vi "MGCC_MdlMgmt_main.vi"() -> ()   [LabVIEW 2016]
doc: "-----------------------------------------------------------------------------------------------------------------------\nCopyright <2019> <The University of Tennessee at Knoxville and the University of Tennessee Research Foundation>\nThis software is released under BSD-3 \nhttps://opensource.org/licenses/BSD-3-Clause \nAdditional license options available at https://utrf.tennessee.edu/industry/sample-agreements/\n-----------------------------------------------------------------------------------------------------------------------\n\nThis VI is the main VI for the model management function. The main purpose of this VI is to initize the input for the state estimation and PQ balancing. Since it will only be run one time, there is no need for the enable button."
uses:
  Communication/MGCC_Global_communication_inputsettings .vi
  Data logging/Sub-Vis/Global tdms reference.vi
  Data logging/Sub-Vis/MGCC_DataLog_global.vi
  Communication/Global communication output.vi
  Communication/Global communication.vi
  Global_MdlMgmt.vi
  Resynchronization/MGCC_Resync_global.vi
  Islanded Control/MGCC_IsdCon_global1.vi
  Abnormal Fault State Control/Sub_VIs/Fault_Abnormal_state.vi
  <vilib>/imath/engines/lvmath2/RunTimeEngine/ErrorHandling/NIMS_Finalize Error.vi
  <vilib>/imath/engines/lvmath2/RunTimeEngine/BuiltInFunctions/double/NIMS_double.vi
  <vilib>/imath/engines/lvmath2/RunTimeEngine/NodeEndStatement/NIMS_NodeEndStatement_Output.vi
panel:
  out "x 2":dbl[][](array[numeric])
  out "x":dbl[][](array[numeric])
  out "appended array":dbl[](array[numeric])
  out "error out 4":errorcluster
  out "error out 3":errorcluster
  out "error out 2":errorcluster
  out "PV_hist":dbl[](array[numeric])
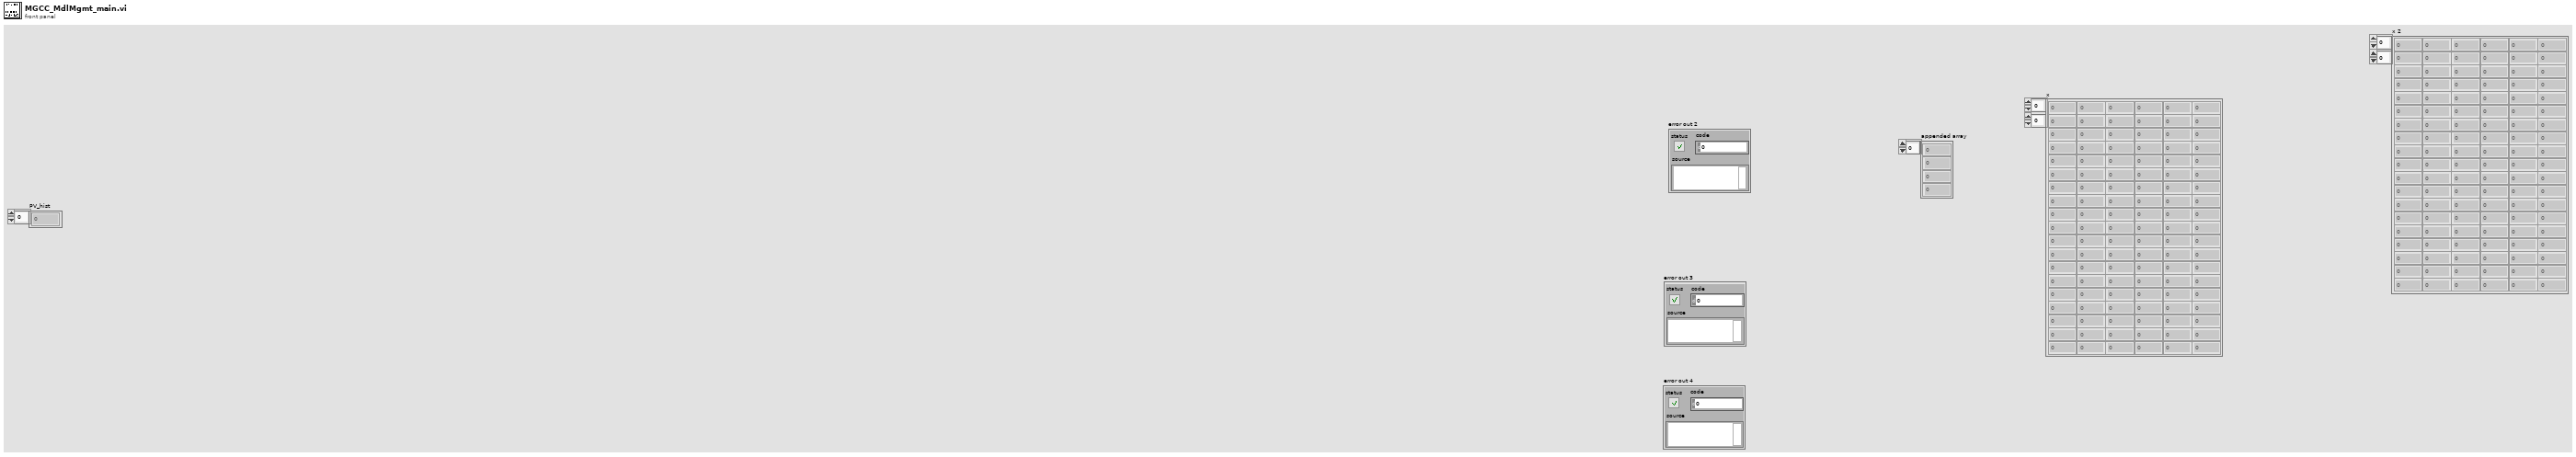
[diagram p1: front panel]
types:
  T1 = enum16{"open", "open or create", "create or replace", "create", "open (read-only)"}
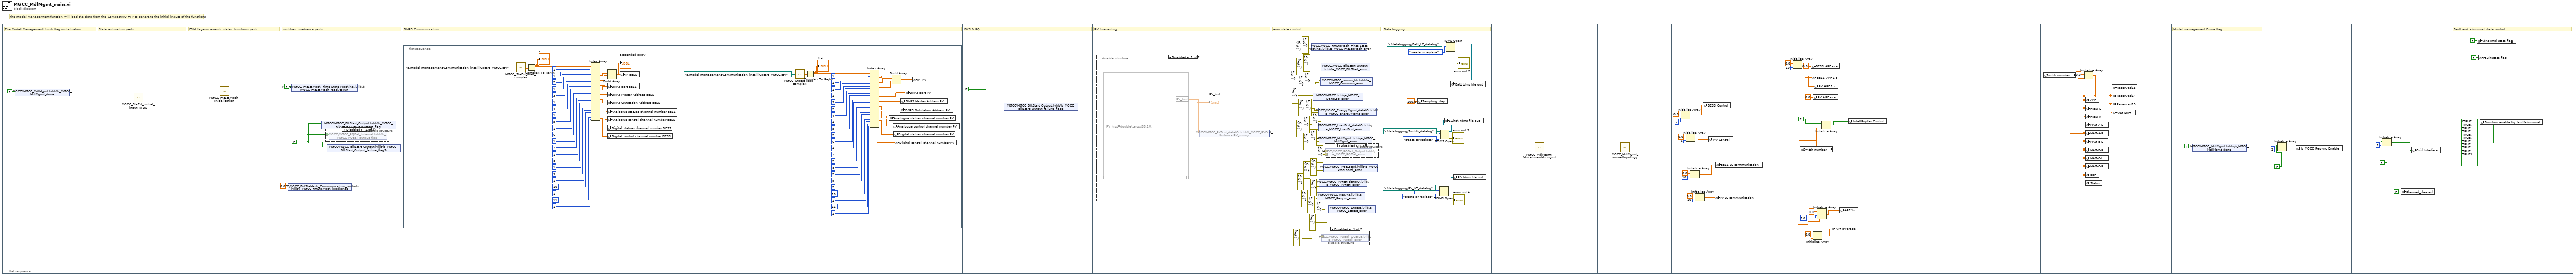
[diagram p0: block diagram]
diagram:
  # "the model management function will load the data from the CompactRIO FTP to generate the initial inputs of the functions"
  n1 = flat-sequence {
    frame #0 {
      # "The Model Management finish flag initialization"
      n2 = shared-variable "MGCC\\MGCC_MdlMgmt.lvlib\\b_MGCC_MdlMgmt_done"(FALSE ("b_MGCC_MdlMgmt_done")) -> ()  [unwired: 1 in, 1 out]
    }
    frame #1 {
      # "State estimation parts"
      n3 = call "MGCC_StaEst_initial_input_RTDS.vi"() -> ()  [unwired: 12 in]
    }
    frame #2 {
      # "FSM flagesm events, states, functions parts"
      n4 = call "MGCC_FntStaMach_Initialization.vi"() -> ()  [unwired: 12 in]
    }
    frame #3 {
      w2 = FALSE ("S0102-status-ctrl")
      # "switches, irradiance parts"
      n5 = shared-variable "MGCC\\MGCC_FntStaMach_Communication_controls.lvlib\\i_MGCC_FntStaMach_irradiance"(0.0 ("i_MGCC_FntStaMach_irradiance")) -> ()  [unwired: 1 in, 1 out]
      n6 = shared-variable "MGCC\\MGCC_FntStaMach_Finte State Machine.lvlib\\b_MGCC_FntStaMach_readytorun"(FALSE ("b_MGCC_FntStaMach_readytorun")) -> ()  [unwired: 1 in, 1 out]
      n7 = shared-variable "MGCC\\MGCC_BlkStart_Output.lvlib\\b_MGCC_BlkStart_Output_success_flag"(w2) -> ()  [unwired: 1 in, 1 out]
      n8 = disable-structure shown="Disabled" {
        disable-tunnel: w2 -> [w5 _]
        frame Disabled {
          n9 = shared-variable "MGCC\\MGCC_PQBal_Internal.lvlib\\b_MGCC_PQBal_output_flag"(w5) -> ()  [unwired: 1 in, 1 out]
        }
        frame Enabled {
        }
      }
      n10 = shared-variable "MGCC\\MGCC_BlkStart_Output.lvlib\\b_MGCC_BlkStart_Output_failure_flag5"(w2) -> ()  [unwired: 1 in, 1 out]
    }
    frame #4 {
      # "DNP3 Communication"
      n11 = flat-sequence {
        frame #0 {
          n12 = call "MGCC_StaEst_load_complex.vi"("file path (dialog if empty)"=path "c:/model-management/Communication_intellirupters_MGCC.csv" ("file path (use dialog)")) -> ("Array 13"=w29:cdb[][])
          n13 = Complex To Re/Im(x + iy=w29) -> (x=w28:dbl[][])  [unwired: 1 out]
          "x" <- w28
          n14 = Index Array(array=w28, index (row) #1=1 ("index (row)"), index (col) #1=1 ("disabled index (col)"), index (row) #2=2 ("index (row)"), index (col) #2=1 ("disabled index (col)"), index (row) #3=3 ("index (row)"), index (col) #3=1 ("disabled index (col)"), index (row) #4=4 ("index (row)"), index (col) #4=1 ("disabled index (col)"), index (row) #5=5 ("index (row)"), index (col) #5=1 ("disabled index (col)"), index (row) #6=6 ("index (row)"), index (col) #6=1 ("disabled index (col)"), index (row) #7=7 ("index (row)"), index (col) #7=1 ("disabled index (col)"), index (row) #8=8 ("index (row)"), index (col) #8=1 ("disabled index (col)"), index (row) #9=9 ("index (row)"), index (col) #9=1 ("disabled index (col)"), index (row) #10=10 ("index (row)"), index (col) #10=1 ("disabled index (col)"), index (row) #11=11 ("index (row)"), index (col) #11=1 ("disabled index (col)")) -> (element #1=w39:dbl, element #2=w32:dbl, element #3=w31:dbl, element #4=w30:dbl, element #5=w12:dbl, element #6=w11:dbl, element #7=w10:dbl, element #8=w9:dbl, element #9=w8:dbl, element #10=w7:dbl, element #11=w6:dbl)
          n15 = Build Array(w39, w32, w31, w30) -> (w13:dbl[])
          "appended array" <- w13
          n16 = global write "MGCC_Global_communication_inputsettings .vi" "DNP3 port BESS"(w12) -> ()
          n17 = global write "MGCC_Global_communication_inputsettings .vi" "DNP3 Master Address BESS"(w11) -> ()
          n18 = global write "MGCC_Global_communication_inputsettings .vi" "DNP3 Outstation Address BESS"(w10) -> ()
          n19 = global write "MGCC_Global_communication_inputsettings .vi" "Analogue statues channel number BESS"(w9) -> ()
          n20 = global write "MGCC_Global_communication_inputsettings .vi" "Analogue control channel number BESS"(w8) -> ()
          n21 = global write "MGCC_Global_communication_inputsettings .vi" "Digital statues channel number BESS"(w7) -> ()
          n22 = global write "MGCC_Global_communication_inputsettings .vi" "Digital control channel number BESS"(w6) -> ()
          n23 = global write "MGCC_Global_communication_inputsettings .vi" "IP_BESS"(w13) -> ()
        }
        frame #1 {
          n24 = call "MGCC_StaEst_load_complex.vi"("file path (dialog if empty)"=path "c:/model-management/Communication_intellirupters_MGCC.csv" ("file path (use dialog)")) -> ("Array 13"=w70:cdb[][])
          n25 = Complex To Re/Im(x + iy=w70) -> (x=w69:dbl[][])  [unwired: 1 out]
          "x 2" <- w69
          n26 = Index Array(array=w69, index (row) #1=1 ("index (row)"), index (col) #1=2 ("disabled index (col)"), index (row) #2=2 ("index (row)"), index (col) #2=2 ("disabled index (col)"), index (row) #3=3 ("index (row)"), index (col) #3=2 ("disabled index (col)"), index (row) #4=4 ("index (row)"), index (col) #4=2 ("disabled index (col)"), index (row) #5=5 ("index (row)"), index (col) #5=2 ("disabled index (col)"), index (row) #6=6 ("index (row)"), index (col) #6=2 ("disabled index (col)"), index (row) #7=7 ("index (row)"), index (col) #7=2 ("disabled index (col)"), index (row) #8=8 ("index (row)"), index (col) #8=2 ("disabled index (col)"), index (row) #9=9 ("index (row)"), index (col) #9=2 ("disabled index (col)"), index (row) #10=10 ("index (row)"), index (col) #10=2 ("disabled index (col)"), index (row) #11=11 ("index (row)"), index (col) #11=2 ("disabled index (col)")) -> (element #1=w54:dbl, element #2=w53:dbl, element #3=w52:dbl, element #4=w51:dbl, element #5=w49:dbl, element #6=w48:dbl, element #7=w47:dbl, element #8=w46:dbl, element #9=w45:dbl, element #10=w44:dbl, element #11=w43:dbl)
          n27 = global write "MGCC_Global_communication_inputsettings .vi" "Analogue statues channel number PV"(w46) -> ()
          n28 = Build Array(w54, w53, w52, w51) -> (w50:dbl[])
          n29 = global write "MGCC_Global_communication_inputsettings .vi" "Analogue control channel number PV"(w45) -> ()
          n30 = global write "MGCC_Global_communication_inputsettings .vi" "Digital statues channel number PV"(w44) -> ()
          n31 = global write "MGCC_Global_communication_inputsettings .vi" "Digital control channel number PV"(w43) -> ()
          n32 = global write "MGCC_Global_communication_inputsettings .vi" "DNP3 Outstation Address PV"(w47) -> ()
          n33 = global write "MGCC_Global_communication_inputsettings .vi" "DNP3 Master Address PV"(w48) -> ()
          n34 = global write "MGCC_Global_communication_inputsettings .vi" "DNP3 port PV"(w49) -> ()
          n35 = global write "MGCC_Global_communication_inputsettings .vi" "IP_PV"(w50) -> ()
        }
      }
    }
    frame #5 {
      # "BKS & PQ"
      n36 = shared-variable "MGCC\\MGCC_BlkStart_Output.lvlib\\b_MGCC_BlkStart_Output_failure_flag5"(FALSE) -> ()  [unwired: 1 in, 1 out]
    }
    frame #6 {
      # "PV forecasting"
      n37 = disable-structure shown="Disabled" {
        frame Disabled {
          n38 = mathscript code="PV_hist=double(zeros(88,1));"() -> ("PV_hist"=w81:dbl[])  [unwired: 1 in, 1 out]
          "PV_hist" <- w81
          n39 = shared-variable "MGCC\\MGCC_PVFcst_dataIO.lvlib\\f_MGCC_PVFcst_HistoricalPV_sunny"(w81) -> ()  [unwired: 1 in, 1 out]
        }
        frame Enabled {
        }
      }
    }
    frame #7 {
      (unwired) errorcluster {"status"=FALSE, "code"=0, "source"=""} ("e_MGCC_Commun_error")
      # "error state control"
      n40 = shared-variable "MGCC\\MGCC_FntStaMach_Finte State Machine.lvlib\\e_MGCC_FntStaMach_Error"(errorcluster {"status"=FALSE, "code"=0, "source"=""} ("e_MGCC_FntStaMach_Error"), error in=errorcluster {"status"=FALSE, "code"=0, "source"=""} ("error in (no error)")) -> ()  [unwired: 1 out]
      n41 = shared-variable "MGCC\\MGCC.lvlib\\e_MGCC_DataLog_error"(errorcluster {"status"=FALSE, "code"=0, "source"=""} ("e_MGCC_DataLog_error"), error in=errorcluster {"status"=FALSE, "code"=0, "source"=""} ("error in (no error)")) -> ()  [unwired: 1 out]
      n42 = shared-variable "MGCC\\MGCC_Resync.lvlib\\e_MGCC_Resync_error"(errorcluster {"status"=FALSE, "code"=0, "source"=""} ("e_MGCC_Resync_error"), error in=errorcluster {"status"=FALSE, "code"=0, "source"=""} ("error in (no error)")) -> ()  [unwired: 1 out]
      n43 = shared-variable "MGCC\\MGCC_EnergyMgmt_dataIO.lvlib\\e_MGCC_EnergyMgmt_error"(errorcluster {"status"=FALSE, "code"=0, "source"=""} ("e_MGCC_EnergyMgmt_error"), error in=errorcluster {"status"=FALSE, "code"=0, "source"=""} ("error in (no error)")) -> ()  [unwired: 1 out]
      n44 = shared-variable "MGCC\\MGCC_LoadFcst_dataIO.lvlib\\e_MGCC_LoadFcst_error"(errorcluster {"status"=FALSE, "code"=0, "source"=""} ("e_MGCC_LoadFcst_error"), error in=errorcluster {"status"=FALSE, "code"=0, "source"=""} ("error in (no error)")) -> ()  [unwired: 1 out]
      n45 = shared-variable "MGCC\\MGCC_MdlMgmt.lvlib\\e_MGCC_MdlMgmt_error"(errorcluster {"status"=FALSE, "code"=0, "source"=""} ("e_MGCC_MdlMgmt_error"), error in=errorcluster {"status"=FALSE, "code"=0, "source"=""} ("error in (no error)")) -> ()  [unwired: 1 out]
      n46 = shared-variable "MGCC\\MGCC_PVFcst_dataIO.lvlib\\e_MGCC_PVFcst_error"(errorcluster {"status"=FALSE, "code"=0, "source"=""} ("e_MGCC_PVFcst_error"), error in=errorcluster {"status"=FALSE, "code"=0, "source"=""} ("error in (no error)")) -> ()  [unwired: 1 out]
      n47 = shared-variable "MGCC\\MGCC_comm_lib.lvlib\\e_MGCC_Commun_error"(errorcluster {"status"=FALSE, "code"=0, "source"=""} ("error in (no error)")) -> ()  [unwired: 1 in, 1 out]
      n48 = shared-variable "MGCC\\MGCC_BlkStart_Output.lvlib\\e_MGCC_BlkStart_error"(errorcluster {"status"=FALSE, "code"=0, "source"=""} ("e_MGCC_BlkStart_error"), error in=errorcluster {"status"=FALSE, "code"=0, "source"=""} ("error in (no error)")) -> ()  [unwired: 1 out]
      n49 = disable-structure shown="Disabled" {
        disable-tunnel: errorcluster {"status"=FALSE, "code"=0, "source"=""} ("e_MGCC_StaEst_error") -> [w123 _]
        frame Disabled {
          n50 = shared-variable "MGCC\\MGCC_PQBal_Output.lvlib\\e_MGCC_PQBal_error"(w123, error in=w123) -> ()  [unwired: 1 out]
        }
        frame Enabled {
        }
      }
      n51 = shared-variable "MGCC\\MGCC_ProtCoord.lvlib\\e_MGCC_ProtCoord_error"(errorcluster {"status"=FALSE, "code"=0, "source"=""} ("e_MGCC_ProtCoord_error"), error in=errorcluster {"status"=FALSE, "code"=0, "source"=""} ("error in (no error)")) -> ()  [unwired: 1 out]
      n52 = disable-structure shown="Disabled" {
        disable-tunnel: errorcluster {"status"=FALSE, "code"=0, "source"=""} ("e_MGCC_PQBal_error") -> [w122 _]
        disable-tunnel: errorcluster {"status"=FALSE, "code"=0, "source"=""} ("error in (no error)") -> [w121 _]
        frame Disabled {
          n53 = shared-variable "MGCC\\MGCC_PQBal_Output.lvlib\\e_MGCC_PQBal_error"(w122, error in=w121) -> ()  [unwired: 1 out]
        }
        frame Enabled {
        }
      }
      n54 = shared-variable "MGCC\\MGCC_StaEst.lvlib\\e_MGCC_StaEst_error"(errorcluster {"status"=FALSE, "code"=0, "source"=""} ("e_MGCC_StaEst_error"), error in=errorcluster {"status"=FALSE, "code"=0, "source"=""} ("error in (no error)")) -> ()  [unwired: 1 out]
    }
    frame #8 {
      # "Data logging"
      n55 = global write "MGCC_DataLog_global.vi" "Sampling step"(100.0 ("Sampling step")) -> ()
      n56 = TDMS Open(10:T1."create or replace" ("operation (0:open)"), 11:path "c:/datalogging/PV_LC_datalog" ("file path (dialog if empty)")) -> (0:→"error out 4":errorcluster, 3:w125:refnum<k34>)  [unwired: 5 in]
      n57 = TDMS Open(10:T1."create or replace" ("operation (0:open)"), 11:path "c:/datalogging/Switch_datalog" ("file path (dialog if empty)")) -> (0:→"error out 3":errorcluster, 3:w129:refnum<k34>)  [unwired: 5 in]
      n58 = global write "Global tdms reference.vi" "Switch tdms file out"(w129) -> ()
      n59 = TDMS Open(10:T1."create or replace" ("operation (0:open)"), 11:path "c:/datalogging/Batt_LC_datalog" ("file path (dialog if empty)")) -> (0:→"error out 2":errorcluster, 3:w133:refnum<k34>)  [unwired: 5 in]
      n60 = global write "Global tdms reference.vi" "Batt tdms file out"(w133) -> ()
      n61 = global write "Global tdms reference.vi" "PV tdms file out"(w125) -> ()
    }
    frame #9 {
      n62 = call "MGCC_MdlMgmt_MovetonewMicrogrid.vi"() -> ()  [unwired: 12 in]
    }
    frame #10 {
      n63 = call "MGCC_MdlMgmt_converttopology.vi"() -> ()  [unwired: 12 in]
    }
    frame #11 {
      n64 = Initialize Array(0.0 ("element"), 7 ("dimension size")) -> (w144:dbl[])
      n65 = Initialize Array(0.0 ("element"), 6 ("dimension size")) -> (w143:dbl[])
      n66 = Initialize Array(0.0 ("element"), 10 ("dimension size")) -> (w138:dbl[])
      n67 = Initialize Array(0.0 ("element"), 10 ("dimension size")) -> (w137:dbl[])
      n68 = global write "Global communication output.vi" "BESS Control"(w144) -> ()
      n69 = global write "Global communication output.vi" "PV Control"(w143) -> ()
      n70 = global write "Global communication.vi" "PV LC communication"(w137) -> ()
      n71 = global write "Global communication.vi" "BESS LC communication"(w138) -> ()
    }
    frame #12 {
      n72 = Initialize Array(0.0 ("element"), 10 ("dimension size")) -> (w151:dbl[])
      n73 = global read "Global_MdlMgmt.vi" "Switch number"() -> (w154:dbl)
      n74 = global write "Global communication.vi" "BESS APF ave"(0.0 ("BESS APF ave")) -> ()
      n75 = global write "Global communication.vi" "BESS APF 1 s"(w151) -> ()
      n76 = global write "Global communication.vi" "PV APF ave"(0.0 ("PV APF ave")) -> ()
      n77 = Initialize Array(0.0 ("element"), w154) -> (w157:dbl[])
      n78 = global write "Global communication.vi" "PV APF 1 s"(w151) -> ()
      n79 = Initialize Array(0.0 ("element"), 10 ("dimension size"), w154) -> (w156:dbl[][])
      n80 = Initialize Array(FALSE, w154) -> (w160:bool[])
      n81 = global write "Global communication.vi" "APF average"(w157) -> ()
      n82 = global write "Global communication.vi" "APF 1s"(w156) -> ()
      n83 = global write "Global communication output.vi" "IntellRupter Control"(w160) -> ()
    }
    frame #13 {
      n84 = global read "Global_MdlMgmt.vi" "Switch number"() -> (w164:dbl)
      n85 = Initialize Array(0.0 ("element"), w164) -> (w162:dbl[])
      n86 = global write "Global communication.vi" "APF"(w162) -> ()
      n87 = global write "Global communication.vi" "FREQ-L"(w162) -> ()
      n88 = global write "Global communication.vi" "FREQ-R"(w162) -> ()
      n89 = global write "Global communication.vi" "MAG-A-L"(w162) -> ()
      n90 = global write "Global communication.vi" "MAG-A-R"(w162) -> ()
      n91 = global write "Global communication.vi" "MAG-B-L"(w162) -> ()
      n92 = global write "Global communication.vi" "MAG-B-R"(w162) -> ()
      n93 = global write "Global communication.vi" "MAG-C-L"(w162) -> ()
      n94 = global write "Global communication.vi" "MAG-C-R"(w162) -> ()
      n95 = global write "Global communication.vi" "RPF"(w162) -> ()
      n96 = global write "Global communication.vi" "Status"(w162) -> ()
      n97 = global write "Global communication.vi" "Reserved13"(w162) -> ()
      n98 = global write "Global communication.vi" "Reserved14"(w162) -> ()
      n99 = global write "Global communication.vi" "Reserved15"(w162) -> ()
      n100 = global write "Global communication.vi" "ANG-DIFF"(w162) -> ()
    }
    frame #14 {
      # "Model management Done flag"
      n101 = shared-variable "MGCC\\MGCC_MdlMgmt.lvlib\\b_MGCC_MdlMgmt_done"(TRUE ("b_MGCC_MdlMgmt_done")) -> ()  [unwired: 1 in, 1 out]
    }
    frame #15 {
      n102 = Initialize Array(FALSE ("b_MGCC_MdlMgmt_done"), 2 ("dimension size")) -> (w168:bool[])
      n103 = global write "MGCC_Resync_global.vi" "b_MGCC_Resync_Enable"(w168) -> ()
    }
    frame #16 {
      n104 = Initialize Array(FALSE ("b_MGCC_MdlMgmt_done"), 2 ("dimension size")) -> (w170:bool[])
      n105 = global write "MGCC_IsdCon_global1.vi" "Planned_cleared"(FALSE ("Planned_cleared")) -> ()
      n106 = global write "MGCC_IsdCon_global1.vi" "Grid Interface"(w170) -> ()
    }
    frame #17 {
      # "Fault and abnormal state control"
      n107 = global write "Fault_Abnormal_state.vi" "Abnormal state flag"(FALSE ("Abnormal state flag")) -> ()
      n108 = global write "Fault_Abnormal_state.vi" "Fault state flag"(FALSE ("Fault state flag")) -> ()
      n109 = global write "Fault_Abnormal_state.vi" "Function enable by fault/abnormal"(bool[] [TRUE, TRUE, TRUE, TRUE, TRUE, TRUE, TRUE, TRUE, TRUE, TRUE, TRUE] ("Function enable by fault/abnormal")) -> ()
    }
  }
